vi "Perform Action.vi"(7 "Instrument":refnum<class "Instrument.lvclass">, 8 "error in":errorcluster, 10 "Input":variant, 11 "Perform Action with Channel DBL Strategy in":refnum<class "Perform Action Remote on Const Channel with DBL Strategy.lvclass">) -> (0 "error out":errorcluster, 2 "Output":variant, 3 "Perform Action with Channel DBL Strategy out":refnum<class "Perform Action Remote on Const Channel with DBL Strategy.lvclass">)   [LabVIEW 2023, in "HAL.lvlib" / "Perform Action Remote on Const Channel with DBL Strategy.lvclass"]
uses:
  Perform Action Remote on Const Channel with DBL Strategy.lvclass
  Perform Action Remote on Const Channel with DBL Strategy.lvclass/Perform Action Remote on Const Channel with DBL Strategy.ctl
  Instrument/Instrument.lvclass
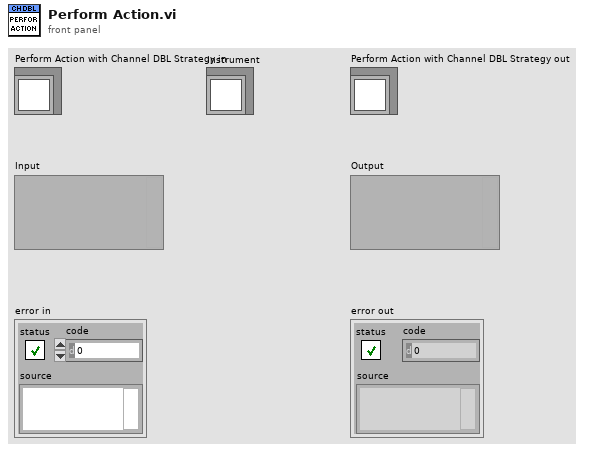
[diagram p1: front panel]
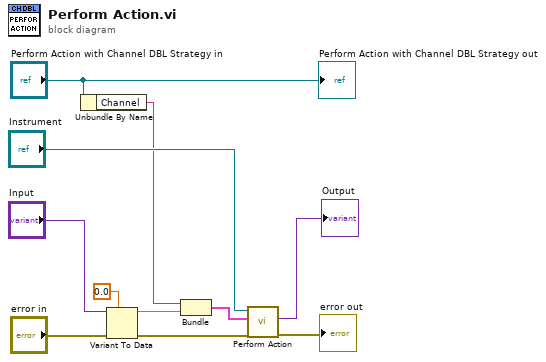
[diagram p0: block diagram]
diagram:
  n1 = Unbundle By Name("Perform Action with Channel DBL Strategy in") -> ("Channel"=w4:string)
  n2 = Variant To Data(error in="error in", type=0.0, Variant="Input") -> (data=w3:dbl, error out=w7:errorcluster)
  n3 = Bundle("Channel"=w4, w3) -> (w2:cluster{"Channel":string, dbl})  [unwired: 1 in]
  n4 = call "Perform Action.vi"("Error In"=w7, "Input"=w2, "reference in"="Instrument") -> ("Error Out"=→"error out":errorcluster, "Output"=→"Output":variant)  [unwired: 6 in, 1 out]
  "Perform Action with Channel DBL Strategy out" <- "Perform Action with Channel DBL Strategy in"
